vi "Semaphore Destroy.vi"(8 "error in (no error)":errorcluster, 11 "Semaphore in":T1) -> (0 "error out":errorcluster, 3 "Semaphore out":T1)   [LabVIEW 2013, in "Linux RT IPC.lvlib" / "POSIX Threads.lvlib" / "Semaphore.lvclass"]
doc: "Calls sem_destroy() on the semaphore object encapsulated by Semaphore.\n\nRefer to online POSIX documentation for more information."
uses:
  Semaphore.lvclass
  Controls/reference.ctl
  POSIX Thread Object/POSIX Thread Object.lvclass/POSIX Thread Object.ctl
  POSIX Thread Object/Private VIs/libpthread path.vi
  POSIX Thread Object/Private VIs/get pthread error.vi
  <vilib>/NI/NI Linux RT Errno/VIs/Public/SubVIs/errno enum to number.vi
  <vilib>/NI/NI Linux RT Errno/VIs/Public/Get Errno Value for Calling Thread.vi
  POSIX Thread Object/POSIX Thread Object.lvclass
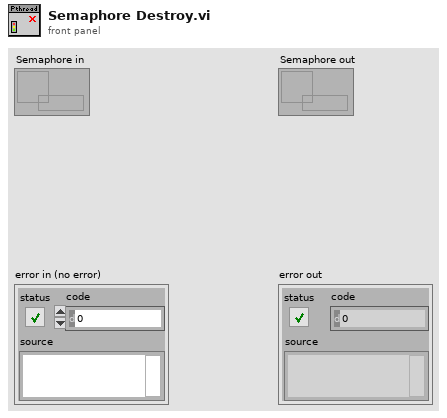
[diagram p1: front panel]
types:
  T1 = typedef "Linux RT IPC.lvlib/POSIX Threads.lvlib/Semaphore.lvclass/reference.ctl" = refnum<data-value>
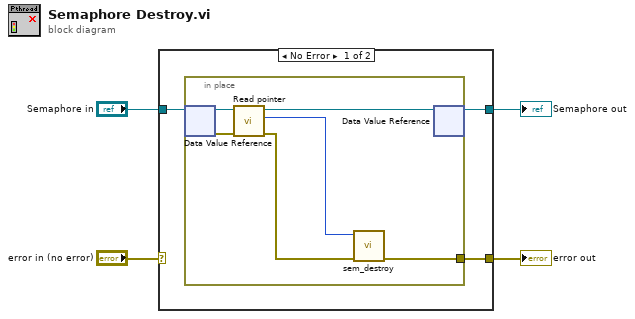
[diagram p0: block diagram]
diagram:
  n1 = case shown="No Error" "error in (no error)" {
    selector: "error in (no error)" -> [_ w14]
    tunnel: "Semaphore in" -> [w7 w15]
    tunnel: [w6 w15] -> w1
    tunnel: [w5 w14] -> w2
    frame No Error {
      n2 = in-place {
        in-place-border: [w10] -> w5
        n3 = in-place-dvr #1(w7) -> (w13:refnum<class "Semaphore.lvclass">, w12:errorcluster)
        n4 = call "Read pointer.vi"("error in (no error)"=w12, "POSIX Thread Object in"=w13) -> ("error out"=w8:errorcluster, "pointer"=w9:u64, "POSIX Thread Object out"=w11:refnum<class "Semaphore.lvclass">)  [unwired: 7 in]
        n5 = call "sem_destroy.vi"("error in (no error)"=w8, "sempahore ptr in"=w9) -> ("error out"=w10:errorcluster)  [unwired: 8 in, 1 out]
        n6 = in-place-dvr #1(w11) -> (w6:T1)  [unwired: 1 out]
      }
    }
    frame Error {
    }
  }
  "error out" <- w2
  "Semaphore out" <- w1
